vi "StableTReached (SubVI).vi"(10 "Numeric":dbl, 11 "Array":dbl[](array[numeric])) -> (2 "Boolean":bool, 3 "mean":dbl)   [LabVIEW 2017, in "Fridge Software v2.1.lvlib"]
uses:
  Fridge Software v2.1.lvlib
  <vilib>/Analysis/baseanly.llb/Mean (DBL).vi
  <vilib>/Analysis/NI_AALBase.lvlib
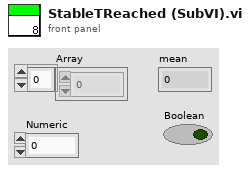
[diagram p1: front panel]
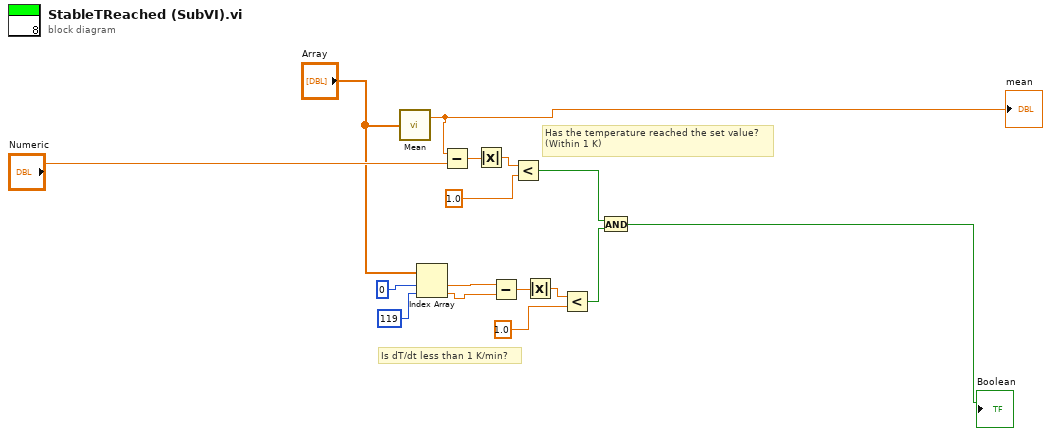
[diagram p0: block diagram]
diagram:
  # "Is dT/dt less than 1 K/min?"
  # "Has the temperature reached the set value?\n(Within 1 K)"
  n1 = call-poly <vilib>:"Mean.vi"("X"="Array") -> ("mean"=w9:dbl)  [unwired: 1 out]
  "mean" <- w9
  n2 = Index Array(array="Array", index #1=0, index #2=119) -> (element #1=w4:dbl, element #2=w5:dbl)
  n3 = Subtract(x=w9, y="Numeric") -> (x-y=w11:dbl)
  n4 = Absolute Value(x=w11) -> (abs(x)=w12:dbl)
  n5 = Subtract(x=w4, y=w5) -> (x-y=w7:dbl)
  n6 = Less?(x=w12, y=1.0) -> (x < y?=w14:bool)
  n7 = Absolute Value(x=w7) -> (abs(x)=w8:dbl)
  n8 = Less?(x=w8, y=1.0) -> (x < y?=w15:bool)
  n9 = And(x=w14, y=w15) -> (x .and. y?=→"Boolean":bool)
